vi "16进制输出.vi"(1 "正常输入":string) -> (0 "16进制输出":string)   [LabVIEW 2018, in "qingshan.lvlib"]
uses:
  qingshan.lvlib
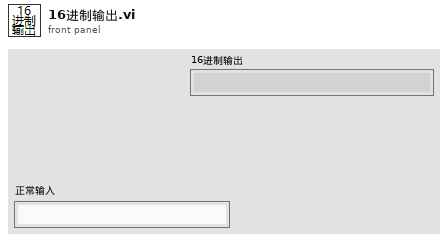
[diagram p1: front panel]
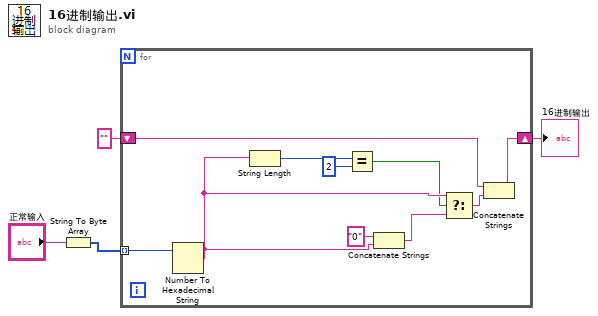
[diagram p0: block diagram]
diagram:
  n1 = String To Byte Array(string="正常输入") -> (unsigned byte array=w3:u8[])
  n2 = for {
    tunnel: w3 -> [w14] mode=indexing
    shift-right: [w5] -> w1
    shift-left: "" -> [w6]
    n3 = Number To Hexadecimal String(2:w14) -> (0:w11:string)  [unwired: 1 in]
    n4 = String Length(string=w11) -> (length=w10:i32)
    n5 = Equal?(x=w10, y=2) -> (x = y?=w8:bool)
    n6 = Concatenate Strings("0" ("字符串"), w11) -> (w12:string)
    n7 = Select(t=w11, s=w8, f=w12) -> (s? t:f=w7:string)
    n8 = Concatenate Strings(w6, w7) -> (w5:string)
  }
  "16进制输出" <- w1
